vi "Gamepad Button Map (n00b).vi"(1 "Joystick Name":string="Right Joystick") -> (0 "Actions":cluster{"STOP MOVING":bool, "n00b Toggle":bool})   [LabVIEW 2012]
uses:
  <vilib>/Rock Robotics/WPI/Joystick/WPI_JoystickGetSetRefNum.vi
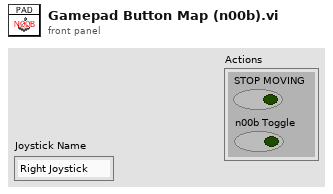
[diagram p1: front panel]
types:
  T1 = typedef "WPI_JoystickDevRef.ctl" = cluster{"Device":T2}
  T2 = typedef "WPI_JoystickDeviceEnum.ctl" = enum16{"USB 1", "USB 2", "USB 3", "USB 4", "Kinect 1", "Kinect 2"}
  T3 = typedef "WPI_JoystickButtonState.ctl" = cluster{"Button 1":bool, "Button 2":bool, "Button 3":bool, "Button 4":bool, "Button 5":bool, "Button 6":bool, "Button 7":bool, "Button 8":bool, "Button 9":bool, "Button 10":bool, "Button 11":bool, "Button 12":bool}
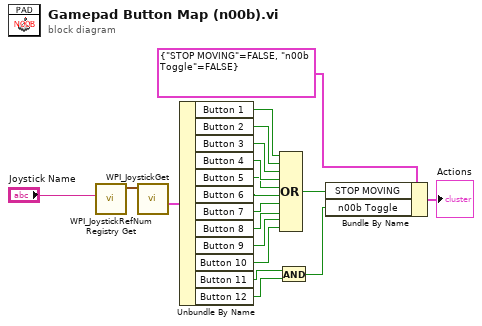
[diagram p0: block diagram]
diagram:
  n1 = call <vilib>:"WPI_JoystickRefNum Registry Get.vi"("refnum name"="Joystick Name") -> ("JoystickDevRef"=w19:T1)  [unwired: 1 in, 9 out]
  n2 = call <vilib>:"WPI_JoystickGet.vi"("JoystickDevRef"=w19) -> ("Buttons"=w17:T3)  [unwired: 1 in, 5 out]
  n3 = Unbundle By Name(w17) -> ("Button 1"=w15:bool, "Button 2"=w14:bool, "Button 3"=w13:bool, "Button 4"=w12:bool, "Button 5"=w11:bool, "Button 6"=w10:bool, "Button 7"=w9:bool, "Button 8"=w8:bool, "Button 9"=w7:bool, "Button 10"=w6:bool, "Button 11"=w4:bool, "Button 12"=w3:bool)
  n4 = And(x=w4, y=w3) -> (x .and. y?=w2:bool)
  n5 = Compound Arithmetic op=OR(w15, w14, w13, w12, w11, w10, w9, w8, w7, w6) -> (w5:bool)
  n6 = Bundle By Name(cluster=cluster{"STOP MOVING":bool, "n00b Toggle":bool} {"STOP MOVING"=FALSE, "n00b Toggle"=FALSE}, "STOP MOVING"=w5, "n00b Toggle"=w2) -> (→"Actions":cluster{"STOP MOVING":bool, "n00b Toggle":bool})
